vi "Actor Core.vi"(8 "error in":errorcluster, 11 "Vision Receiver in":refnum<class "Vision Receiver.lvclass">) -> (0 "error out":errorcluster, 3 "Actor out":refnum<class "Actor.lvclass">)   [LabVIEW 2022 SP3, in "Vision Receiver.lvlib" / "Vision Receiver.lvclass"]
doc: "(<B>Filename</B>: Actor Framework.lvlib:Actor.lvclass:Actor Core.vi)\n\nReceives messages to the actor, reacts to them, and initiates any error handling that may shut the actor down.\n\nDescendant classes may override this VI to append parallel tasks for the actor to complete while it handles messages. Overrides use the Call Parent Class Method node."
uses:
  Vision Receiver.lvclass
  C:/Program Files (x86)/National Instruments/LabVIEW 2022/vi.lib/ActorFramework/Actor/Actor.lvclass
  <vilib>/ActorFramework/Actor/Actor.lvclass
  UDP Reader/UDP Reader/UDP Reader.lvclass
  Vision Receiver.lvclass/Vision Receiver.ctl
  <vilib>/ActorFramework/Actor/Actor.lvclass/Actor.ctl
  <vilib>/ActorFramework/Message Enqueuer/Message Enqueuer.lvclass/Message Enqueuer.ctl
  <vilib>/ActorFramework/Message Enqueuer/Init from Existing Queue.vi
  <vilib>/ActorFramework/Message Enqueuer/Enqueue.vi
  <vilib>/ActorFramework/Stop Msg/Stop Msg.lvclass
  C:/Program Files (x86)/National Instruments/LabVIEW 2022/vi.lib/ActorFramework/Message/Message.lvclass
  <vilib>/ActorFramework/Message Priority Queue/Priority Enqueue.vi
  <vilib>/ActorFramework/Message Enqueuer/Message Enqueuer.lvclass
  <vilib>/MGI/Monitored Actor/Monitored Actor/Monitored Actor/Monitored Actor.lvclass
  C:/Program Files (x86)/National Instruments/LabVIEW 2022/vi.lib/MGI/Monitored Actor/Monitored Actor/Monitored Actor/Monitored Actor.lvclass
  C:/Users/ebert/Documents/codes/ssl/repo/teste/Vision Receiver/Vision Receiver/Vision Receiver.lvclass
  C:/Users/ebert/Documents/codes/ssl/repo/teste/UDP Data Receiver/UDP Data Receiver/UDP Data Receiver.lvclass
  Phoenix/Phoenix Messages/Vision RX Msg/Vision RX Msg.lvclass
panel:
  in  "stop":bool
  out "RX":bool
  out "Data":u8[](array[numeric])
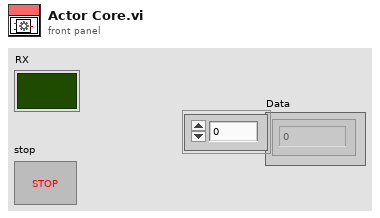
[diagram p1: front panel]
types:
  T1 = cluster{"Stop":refnum<user-event>, "RX":refnum<user-event>}
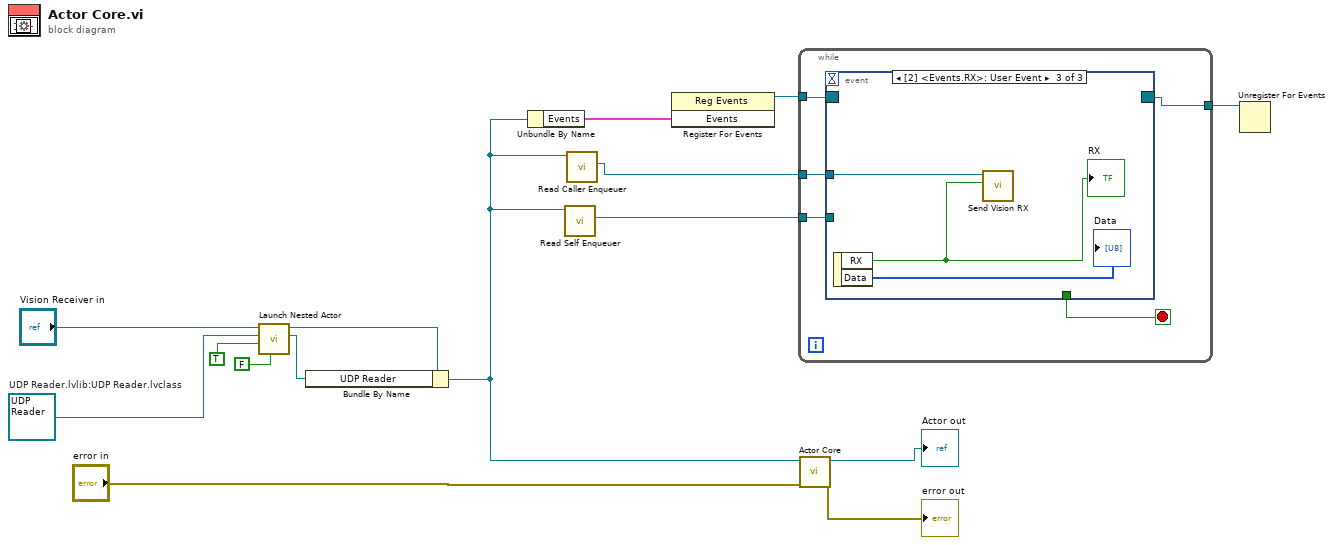
[diagram p0: block diagram]
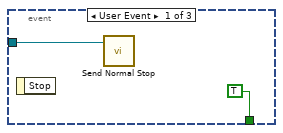
[diagram p2: hidden frame]
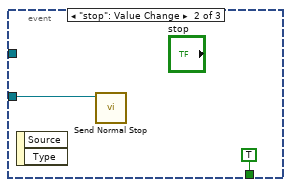
[diagram p3: hidden frame]
diagram:
  w9 = refnum<class "UDP Reader.lvclass"> refnum  # UDP Reader.lvlib:UDP Reader.lvclass
  n1 = call <vilib>:"Launch Nested Actor.vi"("Open Actor Core front panel? (F)"=FALSE, "Auto-stop? (T)"=TRUE, "Nested Actor"=w9, "Caller Actor in"="Vision Receiver in") -> ("Nested Actor's Enqueuer"=w5:refnum<class "Message Enqueuer.lvclass">, "Caller Actor out"=w6:refnum<class "Vision Receiver.lvclass">)  [unwired: 5 in, 1 out]
  n2 = Bundle By Name(cluster=w6, "UDP Reader"=w5) -> (w2:refnum<class "Vision Receiver.lvclass">)
  n3 = Unbundle By Name(w2) -> ("Events"=w10:T1)
  n4 = call <vilib>:"Read Self Enqueuer.vi"("Actor"=w2) -> ("Self Enqueuer"=w4:refnum<class "Message Enqueuer.lvclass">)  [unwired: 10 in]
  n5 = call <vilib>:"Read Caller Enqueuer.vi"("Actor"=w2) -> ("Caller Enqueuer"=w1:refnum<class "Message Enqueuer.lvclass">)  [unwired: 10 in]
  n6 = register-events(w10) -> (reference out=w12:refnum<event-registration>)  [unwired: 2 in, 1 out]
  n7 = while {
    tunnel: w12 -> [w20]
    tunnel: [w19] -> w11
    tunnel: w4 -> [w17]
    tunnel: w1 -> [w16]
    stop <- w18 stop-if-true
    n8 = event shown="[2] <Events.RX>: User Event" {
      selector: w20 -> [_ _ _]
      dyn-events: [_ _ _] -> w19
      timeout: _ -> [_ _ _]
      tunnel: [TRUE TRUE _] -> w18
      tunnel: w17 -> [w21 w23 _]
      tunnel: w16 -> [_ _ w25]
      event User Event {
        n9 = event-data() -> ()  [unwired: 1 in, 1 out]
        n10 = call <vilib>:"Send Normal Stop.vi"("Message Enqueuer"=w21) -> ()  [unwired: 10 in, 1 out]
      }
      event "stop": Value Change {
        n11 = event-data() -> ()  [unwired: 1 in, 2 out]
        n12 = call <vilib>:"Send Normal Stop.vi"("Message Enqueuer"=w23) -> ()  [unwired: 10 in, 1 out]
      }
      event User Event {
        n13 = event-data() -> ("RX"=w26:bool, "Data"=→"Data":u8[])  [unwired: 1 in]
        "RX" <- w26
        n14 = call "Send Vision RX.vi"("RX"=w26, "Message Enqueuer"=w25) -> ()  [unwired: 8 in, 2 out]
      }
    }
  }
  n15 = call-parent "Actor Core.vi"("error in"="error in", "Actor in"=w2) -> ("error out"=→"error out":errorcluster, "Actor out"=→"Actor out":refnum<class "Actor.lvclass">)  [unwired: 8 in]
  n16 = Unregister For Events(event registration refnum=w11) -> ()  [unwired: 1 in, 1 out]
